vi "Finalize.vi"(8 "error in":errorcluster, 11 "Rx UDP Execution Unit in":refnum<class "Rx UDP Execution Unit.lvclass">) -> (0 "error out":errorcluster, 3 "Rx UDP Execution Unit out":refnum<class "Rx UDP Execution Unit.lvclass">)   [LabVIEW 2020, in "AIM ARINC 664 Engine.lvlib" / "Implementation.lvlib" / "Rx UDP Execution Unit.lvclass"]
uses:
  Rx UDP Execution Unit.lvclass
  Program Files/National Instruments/LabVIEW 2025/instr.lib/AIM GmbH/_AIM 664/AIM664LV.lvlib
  Program Files/National Instruments/LabVIEW 2025/instr.lib/AIM GmbH/_AIM 664/bsp/Fdx Stop (Rx).vi
  <vilib>/Utility/SystemLogging/NI_SystemLogging.lvlib
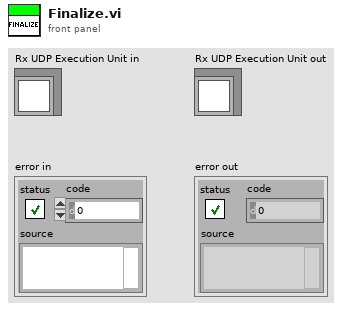
[diagram p1: front panel]
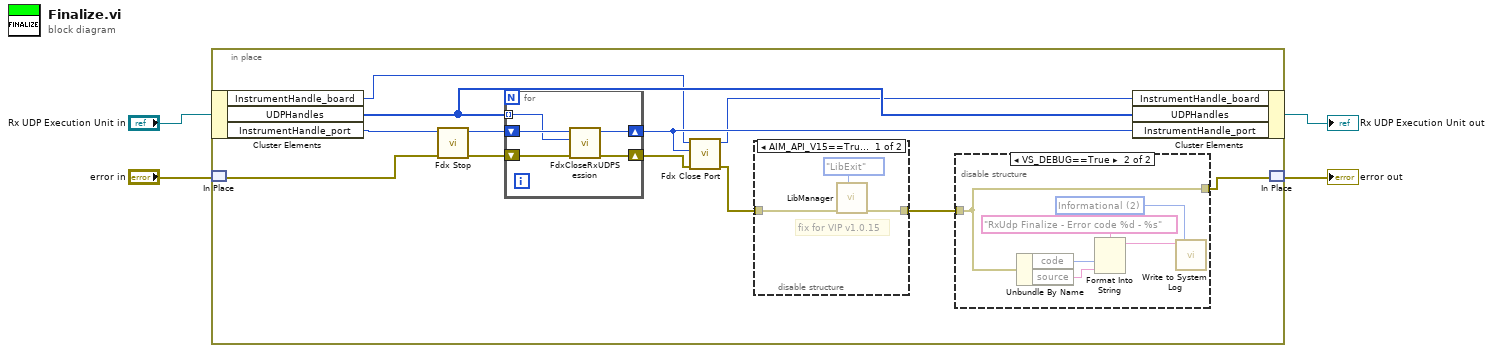
[diagram p0: block diagram]
diagram:
  n1 = in-place {
    n2 = in-place-cluster #1("Rx UDP Execution Unit in") -> ("InstrumentHandle_board"=w9:u32, "UDPHandles"=w12:u32[], "InstrumentHandle_port"=w13:u32)
    n3 = in-place-match #2("error in") -> (w14:errorcluster)
    n4 = call-poly "Fdx Stop.vi"("error in"=w14, "InstrumentHandle_port in"=w13) -> ("error out"=w15:errorcluster, "InstrumentHandle_port out"=w16:u32)  [unwired: 8 in]
    n5 = for {
      shift-right: [w29] -> w10
      shift-left: w16 -> [w32]
      shift-right: [w30] -> w11
      shift-left: w15 -> [w31]
      tunnel: w12 -> [w28] mode=indexing
      n6 = call "FdxCloseRxUDPSession.vi"("error in"=w31, "UdpHandle"=w28, "InstrumentHandle_port"=w32) -> ("error out"=w30:errorcluster, "InstrumentHandle_port"=w29:u32)  [unwired: 7 in]
    }
    n7 = call "Fdx Close Port.vi"("error in"=w11, "InstrumentHandle_port in"=w10, "InstrumentHandle_board in"=w9) -> ("error out"=w6:errorcluster, "InstrumentHandle_board out"=w8:u32)  [unwired: 7 in]
    n8 = disable-structure shown="AIM_API_V15==True" {
      disable-tunnel: w6 -> [w19 w20]
      disable-tunnel: [w18 w20] -> w5
      frame condition #0 {
        # "fix for VIP v1.0.15"
        n9 = call "LibManager.vi"("action"=enum16{"LibInit", "LibExit"}."LibExit", "error in (no error)"=w19) -> ("error out"=w18:errorcluster)  [unwired: 7 in, 2 out]
      }
      frame condition #1 (active) {
      }
    }
    n10 = disable-structure shown="VS_DEBUG==True" {
      disable-tunnel: w5 -> [w21 w22]
      disable-tunnel: [w21 w22] -> w7
      frame condition #0 (active) {
      }
      frame condition #1 {
        w25 = 2 items=["Error", "Warning", "Informational"] ("severity")
        n11 = Unbundle By Name(w22) -> ("code"=w24:i32, "source"=w23:string)
        n12 = Format Into String(format string="RxUdp Finalize - Error code %d - %s", w24, w23) -> (resulting string=w26:string)  [unwired: 2 in, 1 out]
        n13 = call <vilib>:"Write to System Log.vi"("severity"=w25, "message"=w26) -> ()  [unwired: 9 in, 1 out]
      }
    }
    n14 = in-place-cluster #1("InstrumentHandle_board"=w8, "UDPHandles"=w12, "InstrumentHandle_port"=w10) -> (→"Rx UDP Execution Unit out":refnum<class "Rx UDP Execution Unit.lvclass">)
    n15 = in-place-match #2(w7) -> (→"error out":errorcluster)
  }
